vi "Procesamiento Lectura Serial.vi"(11 "Accion":string) -> ()   [LabVIEW 2013, in "Proyecto 2 Touch.lvrbt"]
uses:
  Proyecto 2 Touch.lvrbt
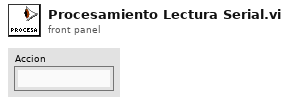
[diagram p1: front panel]
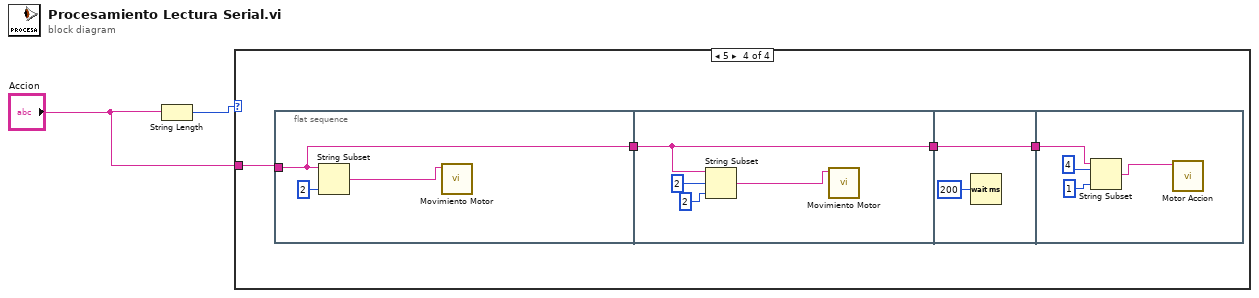
[diagram p0: block diagram]
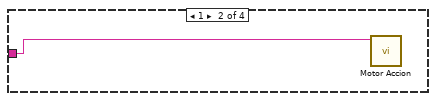
[diagram p3: hidden frame]
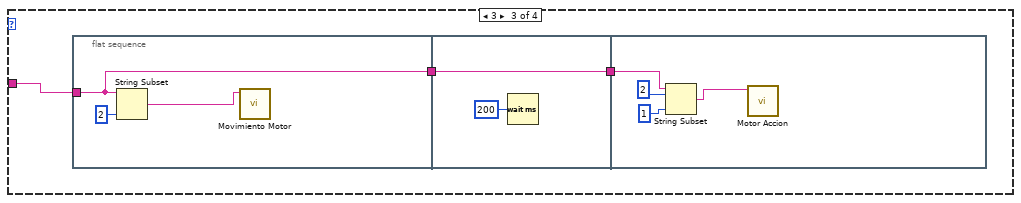
[diagram p4: hidden frame]
diagram:
  n1 = String Length(string="Accion") -> (length=w2:i32)
  n2 = case shown="5" w2 {
    tunnel: "Accion" -> [_ w3 w6 w19]
    frame 0, Default {
    }
    frame 1 {
      n3 = call "Motor Accion.vi"("Tipo Movimiento"=w3) -> ()  [unwired: 11 in]
    }
    frame 3 {
      n4 = flat-sequence {
        tunnel: w6 -> [w7]
        tunnel: [w7] -> w5
        tunnel: w5 -> [w11]
        tunnel: [w11] -> w4
        tunnel: w4 -> [w13]
        frame #0 {
          n5 = String Subset(string=w7, length (rest)=2 ("length (rest)")) -> (substring=w8:string)  [unwired: 1 in]
          n6 = call "Movimiento Motor.vi"("Configuracion Movimiento"=w8) -> ()  [unwired: 11 in]
        }
        frame #1 {
          n7 = Wait (ms)(milliseconds to wait=u32 200) -> ()  [unwired: 1 out]
        }
        frame #2 {
          n8 = String Subset(string=w13, offset (0)=2, length (rest)=1 ("length (rest)")) -> (substring=w12:string)
          n9 = call "Motor Accion.vi"("Tipo Movimiento"=w12) -> ()  [unwired: 11 in]
        }
      }
    }
    frame 5 {
      n10 = flat-sequence {
        tunnel: w19 -> [w20]
        tunnel: [w20] -> w18
        tunnel: w18 -> [w24]
        tunnel: [w24] -> w17
        tunnel: w17 -> [w28]
        tunnel: [w28] -> w16
        tunnel: w16 -> [w30]
        frame #0 {
          n11 = String Subset(string=w20, length (rest)=2 ("length (rest)")) -> (substring=w21:string)  [unwired: 1 in]
          n12 = call "Movimiento Motor.vi"("Configuracion Movimiento"=w21) -> ()  [unwired: 11 in]
        }
        frame #1 {
          n13 = String Subset(string=w24, offset (0)=2, length (rest)=2 ("length (rest)")) -> (substring=w25:string)
          n14 = call "Movimiento Motor.vi"("Configuracion Movimiento"=w25) -> ()  [unwired: 11 in]
        }
        frame #2 {
          n15 = Wait (ms)(milliseconds to wait=u32 200) -> ()  [unwired: 1 out]
        }
        frame #3 {
          n16 = String Subset(string=w30, offset (0)=4, length (rest)=1 ("length (rest)")) -> (substring=w29:string)
          n17 = call "Motor Accion.vi"("Tipo Movimiento"=w29) -> ()  [unwired: 11 in]
        }
      }
    }
  }
